vi "nominal_client.set.vi"(8 "error in (no error)":errorcluster, 10 "Nominal Client.lvclass":refnum<class "Nominal Client.lvclass">, 11 "Multipart Upload in":refnum<class "Multipart Upload.lvclass">) -> (0 "error out":errorcluster, 3 "Multipart Upload out":refnum<class "Multipart Upload.lvclass">)   [LabVIEW 2020, in "Multipart Upload.lvclass"]
uses:
  Multipart Upload.lvclass
  Multipart Upload.lvclass/Multipart Upload.ctl
  Nominal Client/Nominal Client.lvclass
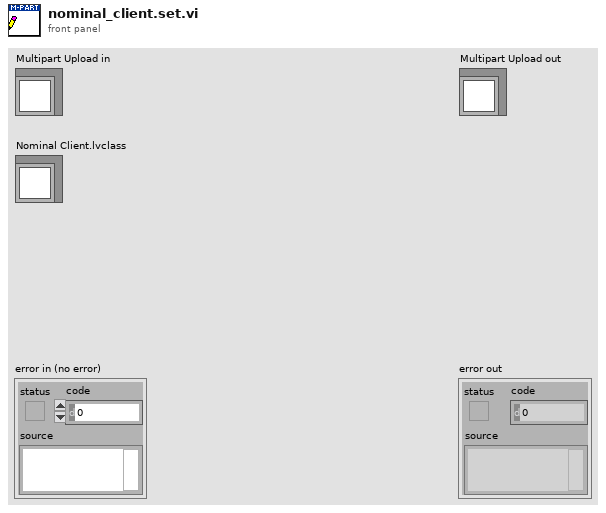
[diagram p1: front panel]
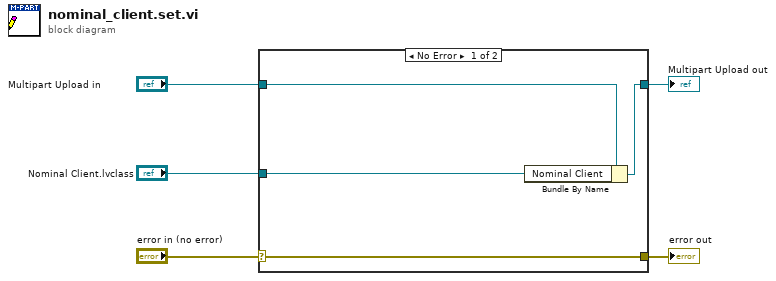
[diagram p0: block diagram]
diagram:
  n1 = case shown="No Error" "error in (no error)" {
    selector: "error in (no error)" -> [w9 w10]
    tunnel: [w9 w10] -> w4
    tunnel: [w7 w11] -> w2
    tunnel: "Multipart Upload in" -> [w8 w11]
    tunnel: "Nominal Client.lvclass" -> [w6 _]
    frame No Error {
      n2 = Bundle By Name(cluster=w8, "Nominal Client"=w6) -> (w7:refnum<class "Multipart Upload.lvclass">)
    }
    frame Error {
    }
  }
  "error out" <- w4
  "Multipart Upload out" <- w2
